vi "AlliGator Variable Names.vi"() -> (0 "Sorted Index Array":i32[](array[numeric]), 1 "Sorted Variable Internal Names":string[](array[string]), 2 "Sorted Basic Variable Names":string[](array[string]), 3 "Basic Variable Names":string[](array[string]))   [LabVIEW 2021, in "AlliGator Phasor Plot.lvlib"]
doc: "Stores basic variable names and their internal counterparts (used in formula)."
uses:
  <userlib>/_OpenG.lib/array/array.llb/Sort 1D Array (I32)__ogtk.vi
  <userlib>/_OpenG.lib/array/array.llb/Reorder 1D Array2 (String)__ogtk.vi
  AlliGator Phasor Plot.lvlib
  <userlib>/_OpenG.lib/array/array.llb/openg_array.lvlib
panel:
  # "see the AlliGator License on the block diagram (Ctrl+E or Window:Show Block Diagram)"
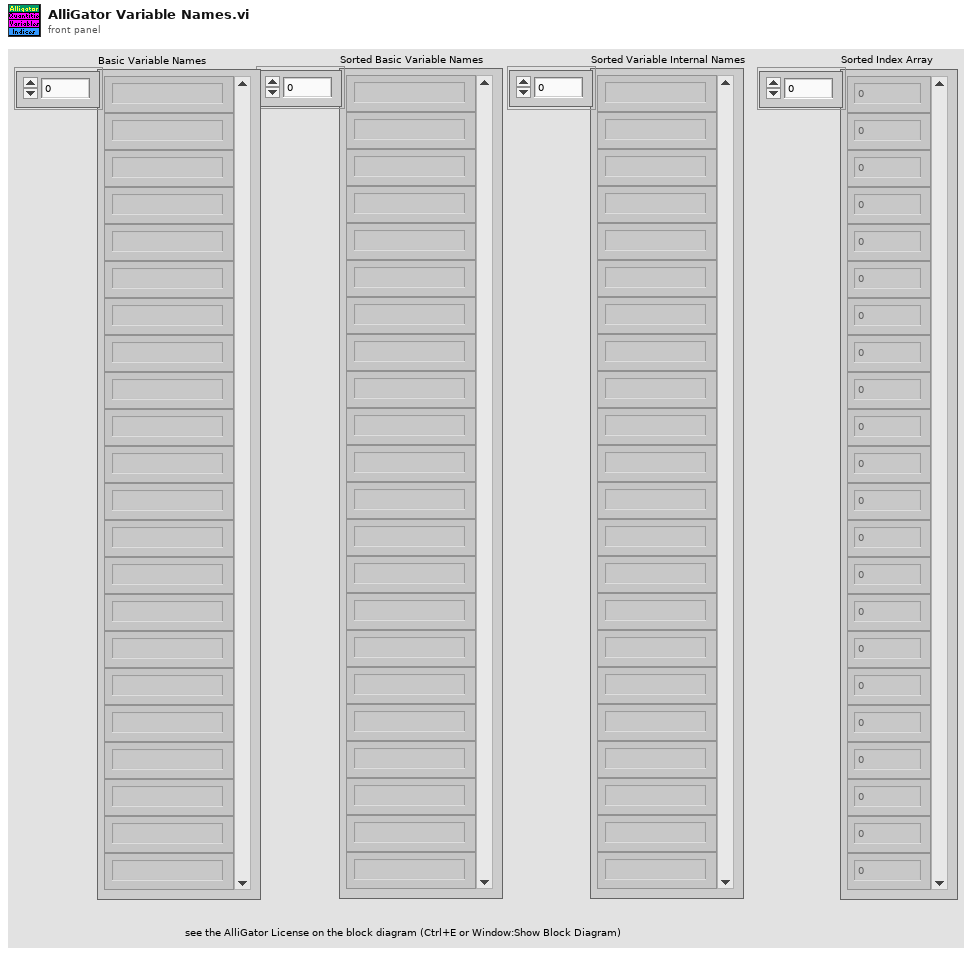
[diagram p1: front panel]
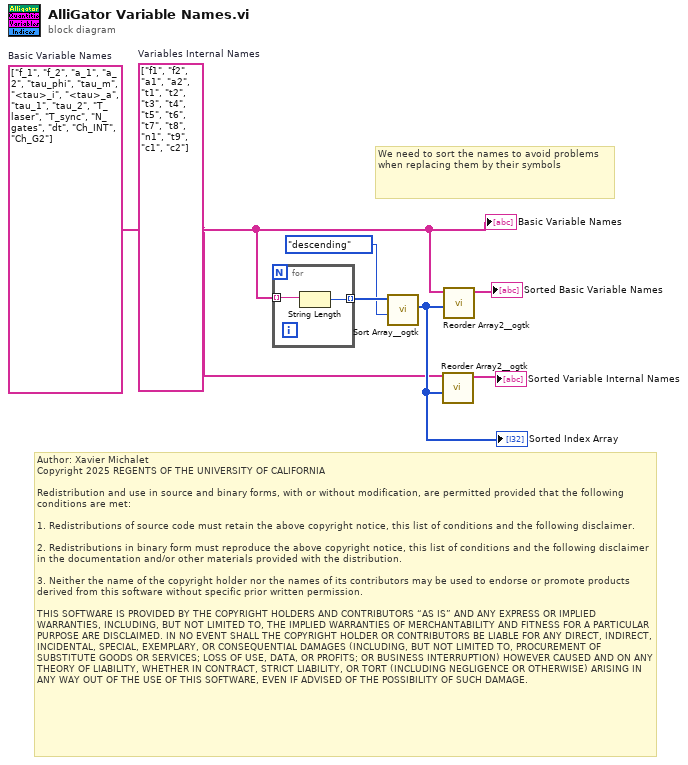
[diagram p0: block diagram]
diagram:
  w1 = string[] ["f1", "f2", "a1", "a2", "t1", "t2", "t3", "t4", "t5", "t6", "t7", "t8", "n1", "t9", "c1", "c2"]  # Variables Internal Names
  w2 = string[] ["f_1", "f_2", "a_1", "a_2", "tau_phi", "tau_m", "<tau>_i", "<tau>_a", "tau_1", "tau_2", "T_laser", "T_sync", "N_gates", "dt", "Ch_INT", "Ch_G2"]  # Basic Variable Names
  # "Author: Xavier Michalet\nCopyright 2025 REGENTS OF THE UNIVERSITY OF CALIFORNIA\n\nRedistribution and use in source and binary forms, with or without modification, are permitted provided that the following conditions are met:\n\n1. Redistributions of source code must retain the above copyright notice, this list of conditions and the following disclaimer.\n\n2. Redistributions in binary form must reproduce the above copyright notice, this list of conditions and the following disclaimer in the documentation and/or other materials provided with the distribution.\n\n3. Neither the name of the copyright holder nor the names of its contributors may be used to endorse or promote products derived from this software without specific prior written permission.\n\nTHIS SOFTWARE IS PROVIDED BY THE COPYRIGHT HOLDERS AND CONTRIBUTORS “AS IS” AND ANY EXPRESS OR IMPLIED WARRANTIES, INCLUDING, BUT NOT LIMITED TO, THE IMPLIED WARRANTIES OF MERCHANTABILITY AND FITNESS FOR A PARTICULAR PURPOSE ARE DISCLAIMED. IN NO EVENT SHALL THE COPYRIGHT HOLDER OR CONTRIBUTORS BE LIABLE FOR ANY DIRECT, INDIRECT, INCIDENTAL, SPECIAL, EXEMPLARY, OR CONSEQUENTIAL DAMAGES (INCLUDING, BUT NOT LIMITED TO, PROCUREMENT OF SUBSTITUTE GOODS OR SERVICES; LOSS OF USE, DATA, OR PROFITS; OR BUSINESS INTERRUPTION) HOWEVER CAUSED AND ON ANY THEORY OF LIABILITY, WHETHER IN CONTRACT, STRICT LIABILITY, OR TORT (INCLUDING NEGLIGENCE OR OTHERWISE) ARISING IN ANY WAY OUT OF THE USE OF THIS SOFTWARE, EVEN IF ADVISED OF THE POSSIBILITY OF SUCH DAMAGE."
  # "We need to sort the names to avoid problems when replacing them by their symbols"
  n1 = for {
    tunnel: w2 -> [w9] mode=indexing
    tunnel: [w8] -> w7 mode=indexing
    n2 = String Length(string=w9) -> (length=w8:i32)
  }
  n3 = call-poly <userlib>:"Sort Array__ogtk.vi"("Order"=enum16{"ascending", "descending"}."descending", "Array in"=w7) -> ("Sorted Pointers"=w3:i32[])  [unwired: 8 in, 1 out]
  "Sorted Index Array" <- w3
  n4 = call-poly <userlib>:"Reorder Array2__ogtk.vi"("indices"=w3, "array"=w1) -> ("reordered array"=→"Sorted Variable Internal Names":string[])  [unwired: 9 in]
  n5 = call-poly <userlib>:"Reorder Array2__ogtk.vi"("indices"=w3, "array"=w2) -> ("reordered array"=→"Sorted Basic Variable Names":string[])  [unwired: 9 in]
  "Basic Variable Names" <- w2
